vi "process_simple_input.vi"(10 "input line":string, 11 "RESP3 Parser in":refnum<class "RESP3 Parser.lvclass">) -> (0 "error out":errorcluster, 2 "value ready?":bool, 3 "RESP3 Parser out":refnum<class "RESP3 Parser.lvclass">, 4 "next bytes":i32)   [LabVIEW 2019, in "RESP3.lvlib" / "RESP3 Parser.lvclass"]
uses:
  RESP3 Parser.lvclass
  RESP3 Parser.lvclass/RESP3 Parser.ctl
  types/RESP3 Type.ctl
  RESP3.lvlib
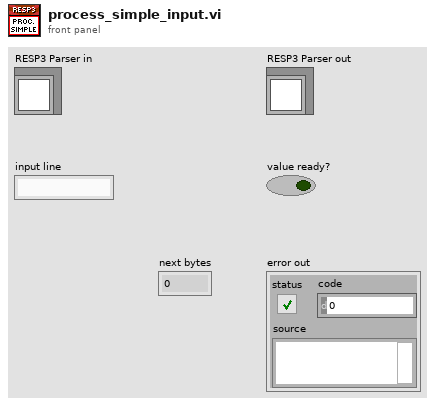
[diagram p1: front panel]
types:
  T1 = typedef "RESP3.lvlib/RESP3 Type.ctl" = enum8{"<0x00>", "<0x01>", "<0x02>", "<0x03>", "<0x04>", "<0x05>", "<0x06>", "<0x07>", "<0x08>", "<0x09>", "<0x0A>", "<0x0B>", "<0x0C>", "<0x0D>", "<0x0E>", "<0x0F>", "<0x10>", "<0x11>", "<0x12>", "<0x13>", "<0x14>", "<0x15>", "<0x16>", "<0x17>", "<0x18>", "<0x19>", "<0x1A>", "<0x1B>", "<0x1C>", "<0x1D>", "<0x1E>", "<0x1F>", "\" \"", "BLOB ERROR", "\"\"\"", "BOOLEAN", "BLOB", "MAP", "\"&\"", "\"'\"", "BIG NUMBER", "\")\"", "ARRAY", "STRING", "DOUBLE", "ERROR", "END", "\"/\"", "\"0\"", "\"1\"", "\"2\"", "\"3\"", "\"4\"", "\"5\"", "\"6\"", "\"7\"", "\"8\"", "\"9\"", "INTEGER", "STREAM", "\"<\"", "VERBATIM STRING", "PUSH", "\"?\"", "\"@\"", "\"A\"", "\"B\"", "\"C\"", "\"D\"", "\"E\"", "\"F\"", "\"G\"", "\"H\"", "\"I\"", "\"J\"", "\"K\"", "\"L\"", "\"M\"", "\"N\"", "\"O\"", "\"P\"", "\"Q\"", "\"R\"", "\"S\"", "\"T\"", "\"U\"", "\"V\"", "\"W\"", "\"X\"", "\"Y\"", "\"Z\"", "\"[\"", "\"\\\"", "\"]\"", "\"^\"", "NULL", "\"`\"", "\"a\"", "\"b\"", "\"c\"", "\"d\"", "\"e\"", "\"f\"", "\"g\"", "\"h\"", "\"i\"", "\"j\"", "\"k\"", "\"l\"", "\"m\"", "\"n\"", "\"o\"", "\"p\"", "\"q\"", "\"r\"", "\"s\"", "\"t\"", "\"u\"", "\"v\"", "\"w\"", "\"x\"", "\"y\"", "\"z\"", "\"{\"", "ATTRIBUTES", "\"}\"", "SET", "<0x7F>", "<0x80>", "<0x81>", "<0x82>", "<0x83>", "<0x84>", "<0x85>", "<0x86>", "<0x87>", "<0x88>", "<0x89>", "<0x8A>", "<0x8B>", "<0x8C>", "<0x8D>", "<0x8E>", "<0x8F>", "<0x90>", "<0x91>", "<0x92>", "<0x93>", "<0x94>", "<0x95>", "<0x96>", "<0x97>", "<0x98>", "<0x99>", "<0x9A>", "<0x9B>", "<0x9C>", "<0x9D>", "<0x9E>", "<0x9F>", "<0xA0>", "<0xA1>", "<0xA2>", "<0xA3>", "<0xA4>", "<0xA5>", "<0xA6>", "<0xA7>", "<0xA8>", "<0xA9>", "<0xAA>", "<0xAB>", "<0xAC>", "<0xAD>", "<0xAE>", "<0xAF>", "<0xB0>", "<0xB1>", "<0xB2>", "<0xB3>", "<0xB4>", "<0xB5>", "<0xB6>", "<0xB7>", "<0xB8>", "<0xB9>", "<0xBA>", "<0xBB>", "<0xBC>", "<0xBD>", "<0xBE>", "<0xBF>", "<0xC0>", "<0xC1>", "<0xC2>", "<0xC3>", "<0xC4>", "<0xC5>", "<0xC6>", "<0xC7>", "<0xC8>", "<0xC9>", "<0xCA>", "<0xCB>", "<0xCC>", "<0xCD>", "<0xCE>", "<0xCF>", "<0xD0>", "<0xD1>", "<0xD2>", "<0xD3>", "<0xD4>", "<0xD5>", "<0xD6>", "<0xD7>", "<0xD8>", "<0xD9>", "<0xDA>", "<0xDB>", "<0xDC>", "<0xDD>", "<0xDE>", "<0xDF>", "<0xE0>", "<0xE1>", "<0xE2>", "<0xE3>", "<0xE4>", "<0xE5>", "<0xE6>", "<0xE7>", "<0xE8>", "<0xE9>", "<0xEA>", "<0xEB>", "<0xEC>", "<0xED>", "<0xEE>", "<0xEF>", "<0xF0>", "<0xF1>", "<0xF2>", "<0xF3>", "<0xF4>", "<0xF5>", "<0xF6>", "<0xF7>", "<0xF8>", "<0xF9>", "<0xFA>", "<0xFB>", "<0xFC>", "<0xFD>", "<0xFE>"}
  T2 = cluster{"index":i32, "remaining elements":i32, "nest type":T1}[]
  T3 = cluster{"index":i32, "remaining elements":i32, "char":T1}[]
  T4 = cluster{"index":i32, "remaining elements":i32, "nest type":T1}
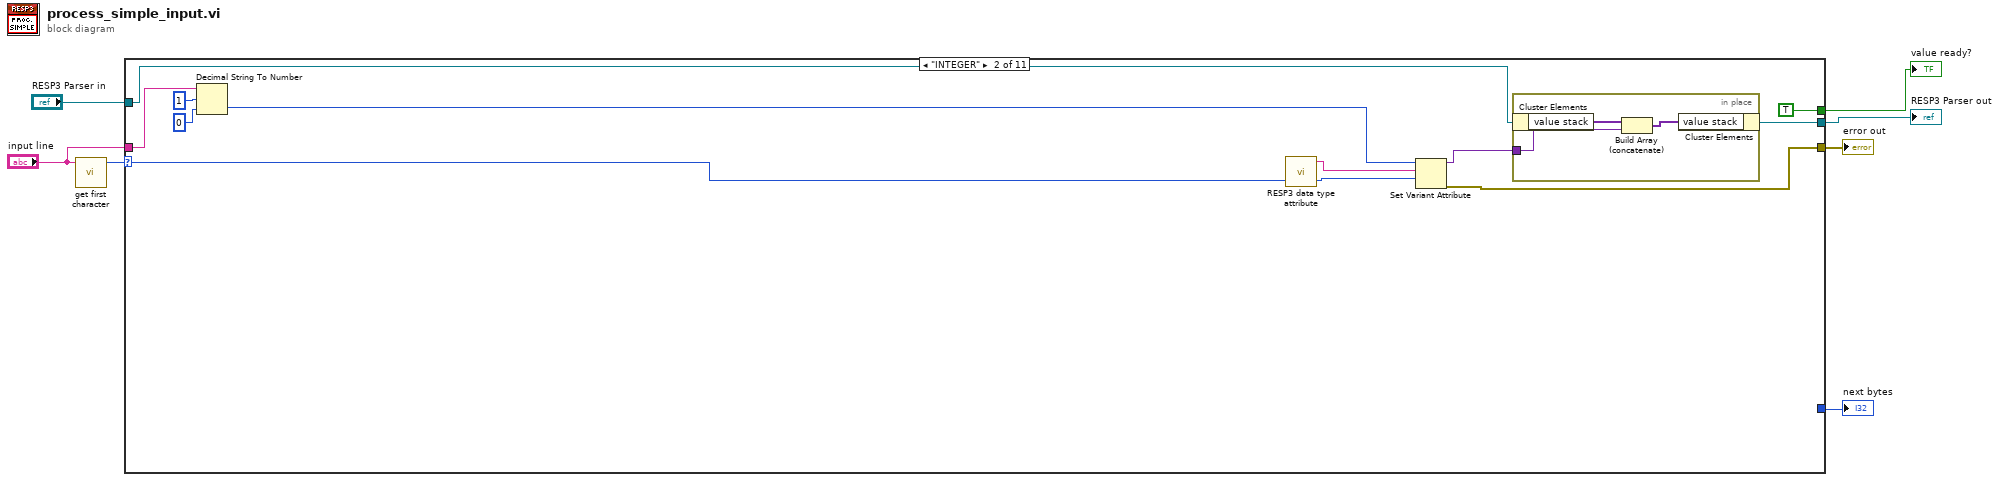
[diagram p0: block diagram]
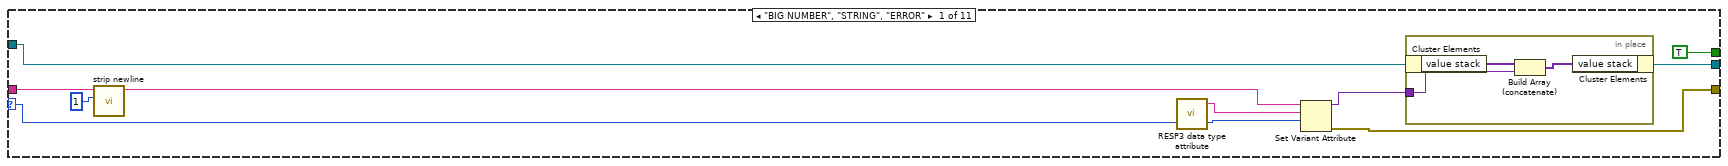
[diagram p2: hidden frame]
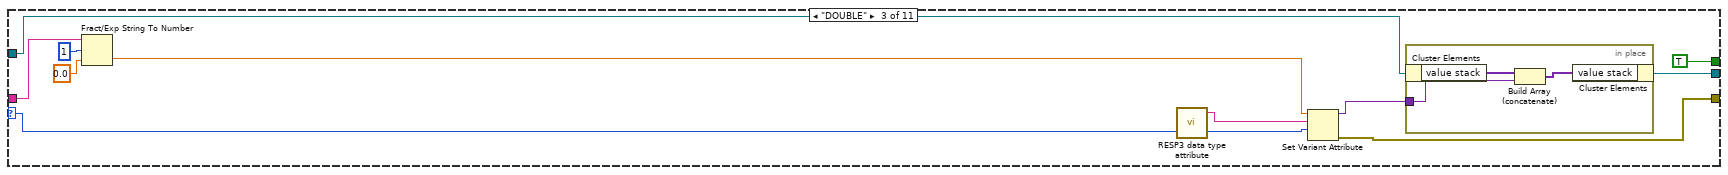
[diagram p3: hidden frame]
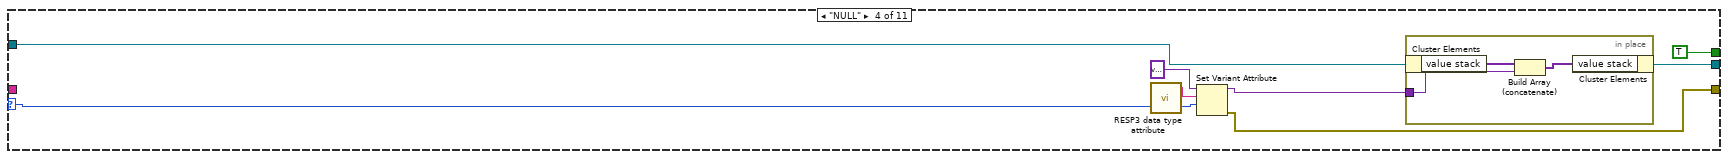
[diagram p4: hidden frame]
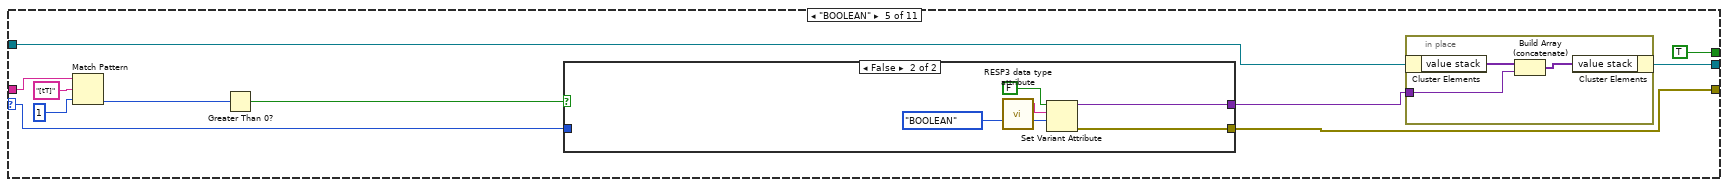
[diagram p5: hidden frame]
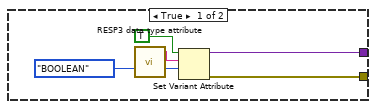
[diagram p6: hidden frame]
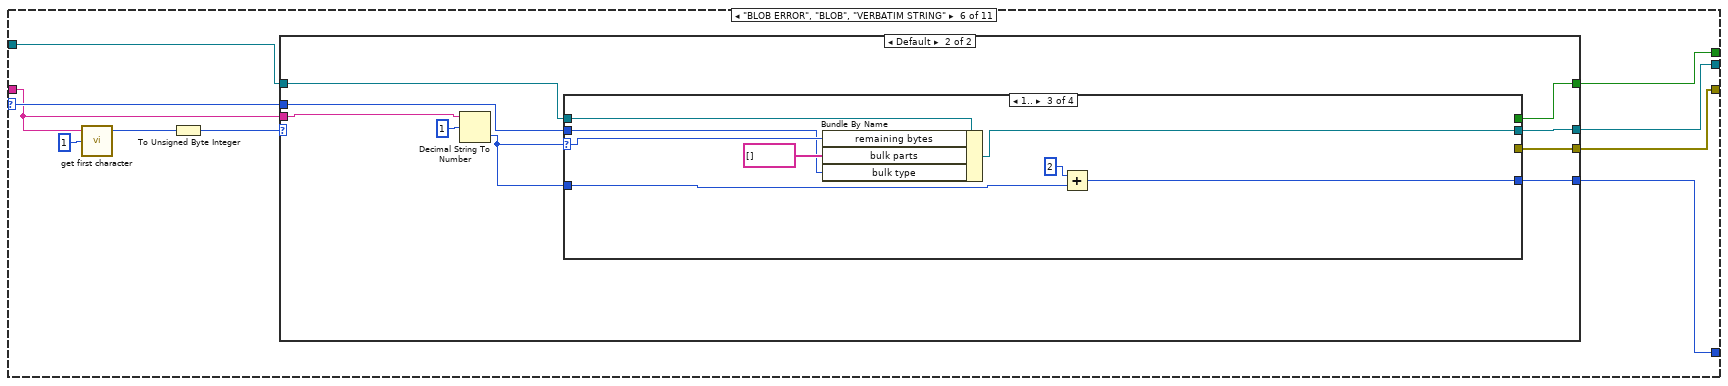
[diagram p7: hidden frame]
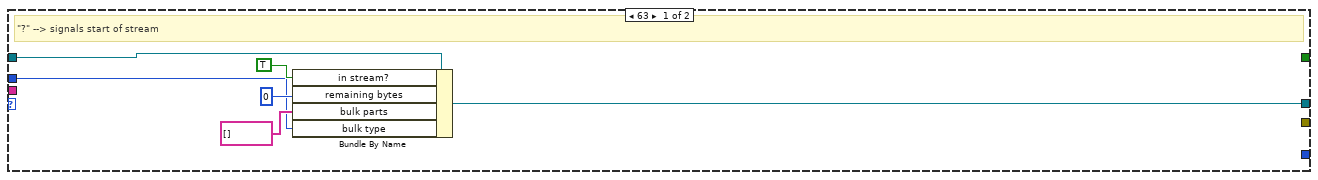
[diagram p8: hidden frame]
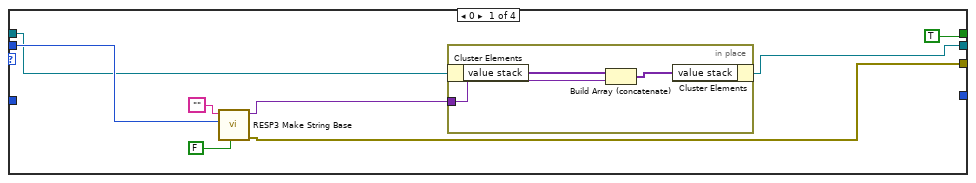
[diagram p9: hidden frame]
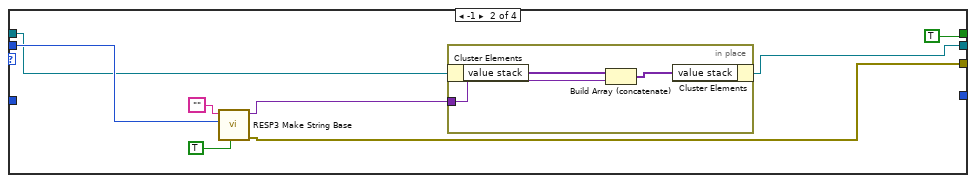
[diagram p10: hidden frame]
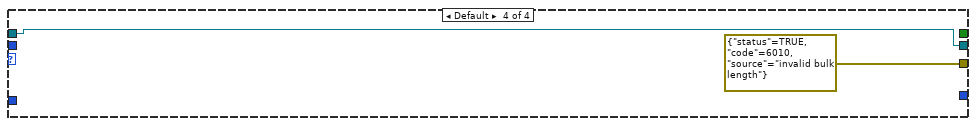
[diagram p11: hidden frame]
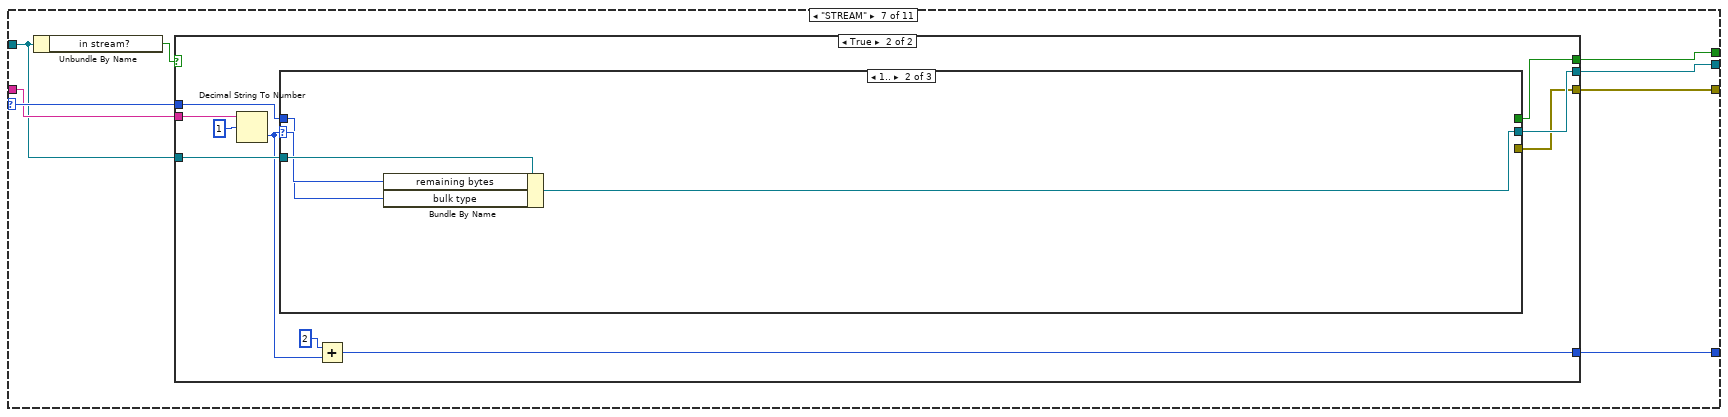
[diagram p12: hidden frame]
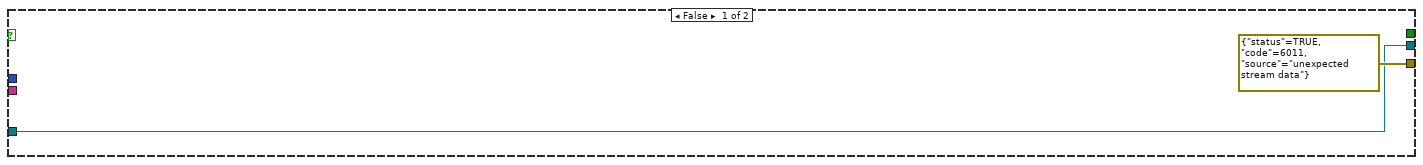
[diagram p13: hidden frame]
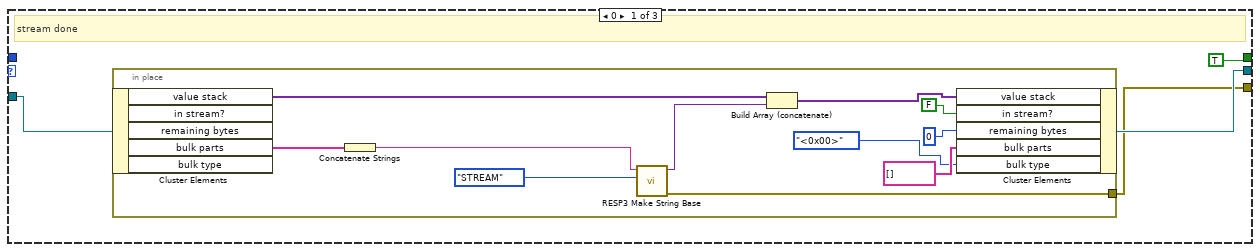
[diagram p14: hidden frame]
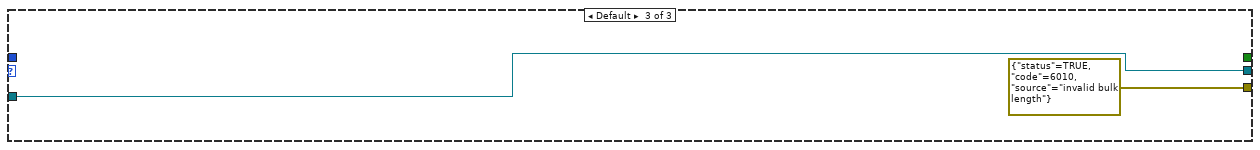
[diagram p15: hidden frame]
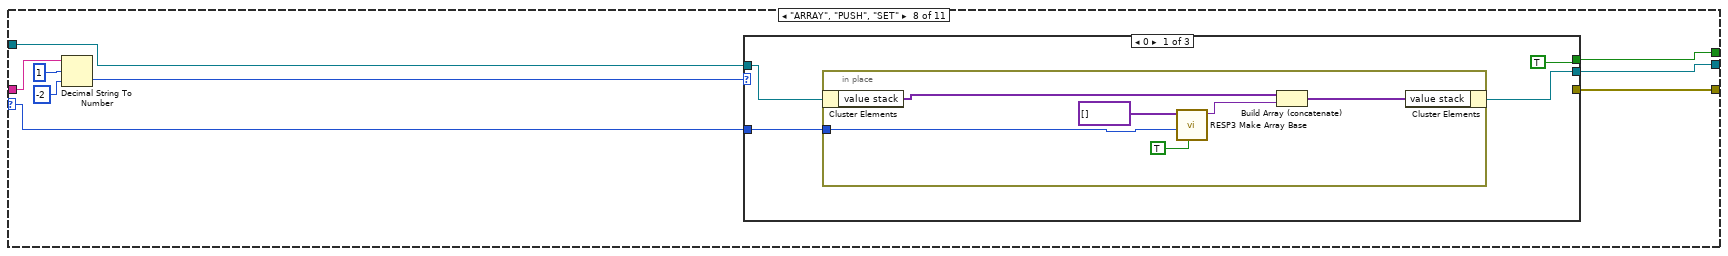
[diagram p16: hidden frame]
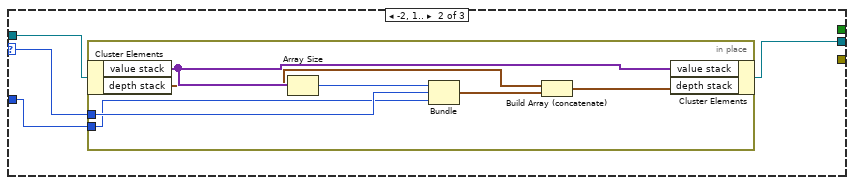
[diagram p17: hidden frame]
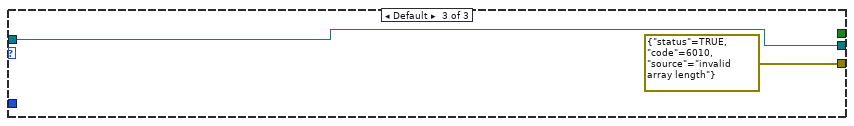
[diagram p18: hidden frame]
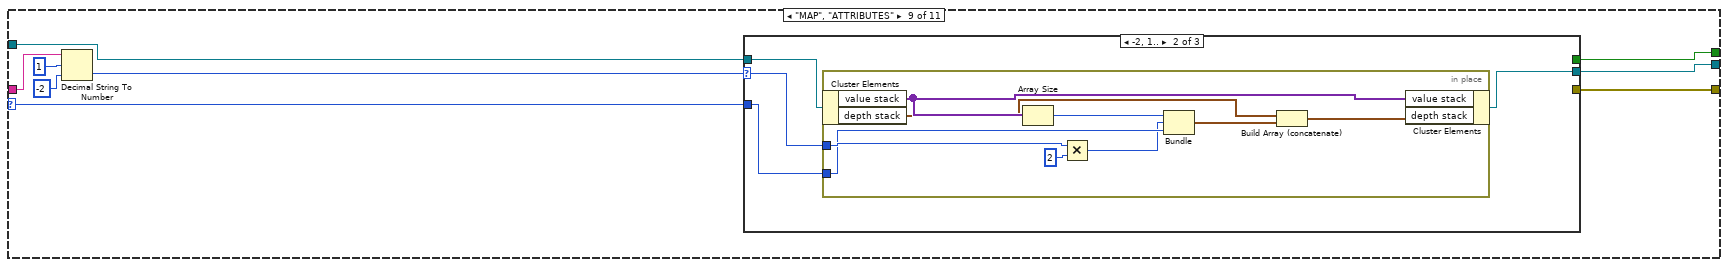
[diagram p19: hidden frame]
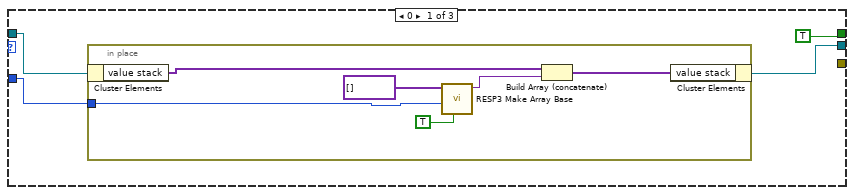
[diagram p20: hidden frame]
diagram:
  n1 = call "get first character.vi"("input"="input line") -> ("char"=w2:T1)  [unwired: 4 in]
  n2 = case shown="\"INTEGER\"" w2 {
    selector: w2 -> [w9 w26 w40 w51 w66 w91 w147 w183 w215 _ _]
    tunnel: "input line" -> [w17 w24 w38 _ w64 w89 w145 w190 w222 _ _]
    tunnel: [TRUE TRUE TRUE TRUE TRUE w85 w144 w185 w217 w249 _] -> w3
    tunnel: "RESP3 Parser in" -> [w14 w30 w44 w55 w69 w93 w143 w188 w220 w250 w265]
    tunnel: [w13 w29 w43 w54 w68 w92 w148 w187 w219 w248 w265] -> w4
    tunnel: [w8 w25 w39 w50 w65 w90 w146 w184 w216 _ _] -> w7
    tunnel: [_ _ _ _ _ w84 w141 _ _ _ _] -> w1
    frame "BIG NUMBER", "STRING", "ERROR" {
      n3 = call "strip newline.vi"("offset"=1, "\\r\\n terminated string"=w17) -> ("striped string"=w12:string)  [unwired: 9 in]
      n4 = call "RESP3 data type attribute.vi"() -> ("dt attribute"=w10:string)  [unwired: 5 in]
      n5 = Set Variant Attribute(Variant=w12, name=w10, value=w9) -> (Variant out=w11:variant, error out=w8:errorcluster)  [unwired: 1 in, 1 out]
      n6 = in-place {
        in-place-border: w11 -> [w19]
        n7 = in-place-cluster #1(w14) -> ("value stack"=w20:variant[])
        n8 = Build Array (concatenate)(w20, w19) -> (w18:variant[])
        n9 = in-place-cluster #1("value stack"=w18) -> (w13:refnum<class "RESP3 Parser.lvclass">)
      }
    }
    frame "INTEGER" {
      n10 = Decimal String To Number(string=w24, offset=1, default (0L)=i64 0 ("default (0 I32)")) -> (number=w21:i64)  [unwired: 1 out]
      n11 = call "RESP3 data type attribute.vi"() -> ("dt attribute"=w27:string)  [unwired: 5 in]
      n12 = Set Variant Attribute(Variant=w21, name=w27, value=w26) -> (Variant out=w28:variant, error out=w25:errorcluster)  [unwired: 1 in, 1 out]
      n13 = in-place {
        in-place-border: w28 -> [w33]
        n14 = in-place-cluster #2(w30) -> ("value stack"=w34:variant[])
        n15 = Build Array (concatenate)(w34, w33) -> (w32:variant[])
        n16 = in-place-cluster #2("value stack"=w32) -> (w29:refnum<class "RESP3 Parser.lvclass">)
      }
    }
    frame "DOUBLE" {
      n17 = Fract/Exp String To Number(string=w38, offset=1, default (0 dbl)=0.0 ("default (0 I32)")) -> (number=w35:dbl)  [unwired: 1 in, 1 out]
      n18 = call "RESP3 data type attribute.vi"() -> ("dt attribute"=w41:string)  [unwired: 5 in]
      n19 = Set Variant Attribute(Variant=w35, name=w41, value=w40) -> (Variant out=w42:variant, error out=w39:errorcluster)  [unwired: 1 in, 1 out]
      n20 = in-place {
        in-place-border: w42 -> [w47]
        n21 = in-place-cluster #3(w44) -> ("value stack"=w48:variant[])
        n22 = Build Array (concatenate)(w48, w47) -> (w46:variant[])
        n23 = in-place-cluster #3("value stack"=w46) -> (w43:refnum<class "RESP3 Parser.lvclass">)
      }
    }
    frame "NULL" {
      n24 = call "RESP3 data type attribute.vi"() -> ("dt attribute"=w52:string)  [unwired: 5 in]
      n25 = Set Variant Attribute(Variant=variant, name=w52, value=w51) -> (Variant out=w53:variant, error out=w50:errorcluster)  [unwired: 1 in, 1 out]
      n26 = in-place {
        in-place-border: w53 -> [w58]
        n27 = in-place-cluster #4(w55) -> ("value stack"=w59:variant[])
        n28 = Build Array (concatenate)(w59, w58) -> (w57:variant[])
        n29 = in-place-cluster #4("value stack"=w57) -> (w54:refnum<class "RESP3 Parser.lvclass">)
      }
    }
    frame "BOOLEAN" {
      n30 = Match Pattern(string=w64, regular expression="[tT]", offset (0)=1) -> (offset past match=w61:i32)  [unwired: 3 out]
      n31 = Greater Than 0?(x=w61) -> (x > 0?=w60:bool)
      n32 = case shown="False" w60 {
        tunnel: [w75 w80] -> w67
        tunnel: w66 -> [_ _]
        tunnel: [w73 w78] -> w65
        frame True {
          n33 = call "RESP3 data type attribute.vi"() -> ("dt attribute"=w74:string)  [unwired: 5 in]
          n34 = Set Variant Attribute(Variant=TRUE, name=w74, value=RESP3_Type."BOOLEAN" ("char")) -> (Variant out=w75:variant, error out=w73:errorcluster)  [unwired: 1 in, 1 out]
        }
        frame False {
          n35 = call "RESP3 data type attribute.vi"() -> ("dt attribute"=w79:string)  [unwired: 5 in]
          n36 = Set Variant Attribute(Variant=FALSE, name=w79, value=RESP3_Type."BOOLEAN" ("char")) -> (Variant out=w80:variant, error out=w78:errorcluster)  [unwired: 1 in, 1 out]
        }
      }
      n37 = in-place {
        in-place-border: w67 -> [w82]
        n38 = in-place-cluster #5(w69) -> ("value stack"=w83:variant[])
        n39 = Build Array (concatenate)(w83, w82) -> (w81:variant[])
        n40 = in-place-cluster #5("value stack"=w81) -> (w68:refnum<class "RESP3 Parser.lvclass">)
      }
    }
    frame "BLOB ERROR", "BLOB", "VERBATIM STRING" {
      n41 = call "get first character.vi"("index"=1, "input"=w89) -> ("char"=w87:T1)  [unwired: 3 in]
      n42 = To Unsigned Byte Integer(number=w87) -> (unsigned 8bit integer=w86:u8)
      n43 = case shown="Default" w86 {
        tunnel: w93 -> [w99 w107]
        tunnel: [w98 w106] -> w92
        tunnel: w91 -> [w94 w105]
        tunnel: [_ w104] -> w90
        tunnel: w89 -> [_ w103]
        tunnel: [_ w102] -> w85
        tunnel: [_ w100] -> w84
        frame 63 {
          # "\"?\" --> signals start of stream"
          n44 = Bundle By Name(cluster=w99, "in stream?"=TRUE ("bulk data.in stream?"), "remaining bytes"=0 ("bulk data.remaining bytes"), "bulk parts"=string[] [] ("bulk data.bulk parts"), "bulk type"=w94) -> (w98:refnum<class "RESP3 Parser.lvclass">)
        }
        frame Default {
          n45 = Decimal String To Number(string=w103, offset=1) -> (number=w101:i32)  [unwired: 1 in, 1 out]
          n46 = case shown="1.." w101 {
            selector: w101 -> [_ _ w135 _]
            tunnel: w107 -> [w113 w124 w137 w139]
            tunnel: [w116 w127 w136 w139] -> w106
            tunnel: w105 -> [w115 w126 w134 _]
            tunnel: [w114 w125 _ errorcluster {"status"=TRUE, "code"=6010, "source"="invalid bulk length"} ("error out")] -> w104
            tunnel: [TRUE TRUE _ _] -> w102
            tunnel: w101 -> [_ _ w133 _]
            tunnel: [_ _ w131 _] -> w100
            frame 0 {
              n47 = call "RESP3 Make String Base.vi"("is null?"=FALSE, "RESP3 String Type"=w115, "string in"="") -> ("error out"=w114:errorcluster, "RESP3 Value out"=w109:variant)  [unwired: 7 in]
              n48 = in-place {
                in-place-border: w109 -> [w117]
                n49 = in-place-cluster #6(w113) -> ("value stack"=w119:variant[])
                n50 = Build Array (concatenate)(w119, w117) -> (w118:variant[])
                n51 = in-place-cluster #6("value stack"=w118) -> (w116:refnum<class "RESP3 Parser.lvclass">)
              }
            }
            frame -1 {
              n52 = call "RESP3 Make String Base.vi"("is null?"=TRUE, "RESP3 String Type"=w126, "string in"="") -> ("error out"=w125:errorcluster, "RESP3 Value out"=w120:variant)  [unwired: 7 in]
              n53 = in-place {
                in-place-border: w120 -> [w128]
                n54 = in-place-cluster #7(w124) -> ("value stack"=w130:variant[])
                n55 = Build Array (concatenate)(w130, w128) -> (w129:variant[])
                n56 = in-place-cluster #7("value stack"=w129) -> (w127:refnum<class "RESP3 Parser.lvclass">)
              }
            }
            frame 1.. {
              n57 = Bundle By Name(cluster=w137, "remaining bytes"=w135, "bulk parts"=string[] [] ("bulk data.bulk parts"), "bulk type"=w134) -> (w136:refnum<class "RESP3 Parser.lvclass">)
              n58 = Add(x=2, y=w133) -> (x+y=w131:i32)
            }
            frame Default {
            }
          }
        }
      }
    }
    frame "STREAM" {
      n59 = Unbundle By Name(w143) -> ("in stream?"=w142:bool)
      n60 = case shown="True" w142 {
        tunnel: [w149 w160] -> w148
        tunnel: w147 -> [_ w159]
        tunnel: [errorcluster {"status"=TRUE, "code"=6011, "source"="unexpected stream data"} ("error out") w158] -> w146
        tunnel: w145 -> [_ w157]
        tunnel: [_ w156] -> w144
        tunnel: w143 -> [w149 w154]
        tunnel: [_ w152] -> w141
        frame False {
        }
        frame True {
          n61 = Decimal String To Number(string=w157, offset=1) -> (number=w153:i32)  [unwired: 1 in, 1 out]
          n62 = case shown="1.." w153 {
            selector: w153 -> [_ w177 _]
            tunnel: w154 -> [w163 w179 w180]
            tunnel: [w162 w178 w180] -> w160
            tunnel: w159 -> [_ w176 _]
            tunnel: [w161 _ errorcluster {"status"=TRUE, "code"=6010, "source"="invalid bulk length"} ("error out")] -> w158
            tunnel: [TRUE _ _] -> w156
            frame 0 {
              # "stream done"
              n63 = in-place {
                in-place-border: [w165] -> w161
                n64 = in-place-cluster #8(w163) -> ("value stack"=w175:variant[], "bulk parts"=w167:string[])  [unwired: 3 out]
                n65 = Concatenate Strings(w167) -> (w166:string)
                n66 = call "RESP3 Make String Base.vi"("RESP3 String Type"=RESP3_Type."STREAM", "string in"=w166) -> ("error out"=w165:errorcluster, "RESP3 Value out"=w173:variant)  [unwired: 8 in]
                n67 = Build Array (concatenate)(w175, w173) -> (w174:variant[])
                n68 = in-place-cluster #8("value stack"=w174, "in stream?"=FALSE ("bulk data.in stream?"), "remaining bytes"=0 ("bulk data.remaining bytes"), "bulk parts"=string[] [] ("bulk data.bulk parts"), "bulk type"=RESP3_Type."<0x00>" ("bulk data.bulk type")) -> (w162:refnum<class "RESP3 Parser.lvclass">)
              }
            }
            frame 1.. {
              n69 = Bundle By Name(cluster=w179, "remaining bytes"=w177, "bulk type"=w176) -> (w178:refnum<class "RESP3 Parser.lvclass">)
            }
            frame Default {
            }
          }
          n70 = Add(x=2, y=w153) -> (x+y=w152:i32)
        }
      }
    }
    frame "ARRAY", "PUSH", "SET" {
      n71 = Decimal String To Number(string=w190, offset=1, default (0L)=-2 ("default (0 I32)")) -> (number=w186:i32)  [unwired: 1 out]
      n72 = case shown="0" w186 {
        selector: w186 -> [_ w202 _]
        tunnel: w188 -> [w194 w204 w213]
        tunnel: [w193 w203 w213] -> w187
        tunnel: [TRUE _ _] -> w185
        tunnel: [_ _ errorcluster {"status"=TRUE, "code"=6010, "source"="invalid array length"} ("error out")] -> w184
        tunnel: w183 -> [w191 w201 _]
        frame 0 {
          n73 = in-place {
            in-place-border: w191 -> [w195]
            n74 = in-place-cluster #9(w194) -> ("value stack"=w200:variant[])
            n75 = call "RESP3 Make Array Base.vi"("is null?"=TRUE, "RESP3 Type"=w195, "RESP3 Values in"=variant[] []) -> ("RESP3 Value out"=w196:variant)  [unwired: 7 in, 1 out]
            n76 = Build Array (concatenate)(w200, w196) -> (w199:variant[])
            n77 = in-place-cluster #9("value stack"=w199) -> (w193:refnum<class "RESP3 Parser.lvclass">)
          }
        }
        frame -2, 1.. {
          n78 = in-place {
            in-place-border: w202 -> [w207]
            in-place-border: w201 -> [w205]
            n79 = in-place-cluster #10(w204) -> ("value stack"=w211:variant[], "depth stack"=w210:T2)
            n80 = Array Size(array=w211) -> (size(s)=w208:i32)
            n81 = Bundle(w208, w207, "char"=w205) -> (w206:cluster{i32, i32, "char":T1})  [unwired: 1 in]
            n82 = Build Array (concatenate)(w210, w206) -> (w209:T3)
            n83 = in-place-cluster #10("value stack"=w211, "depth stack"=w209) -> (w203:refnum<class "RESP3 Parser.lvclass">)
          }
        }
        frame Default {
        }
      }
    }
    frame "MAP", "ATTRIBUTES" {
      n84 = Decimal String To Number(string=w222, offset=1, default (0L)=-2 ("default (0 I32)")) -> (number=w218:i32)  [unwired: 1 out]
      n85 = case shown="-2, 1.." w218 {
        selector: w218 -> [_ w234 _]
        tunnel: w220 -> [w226 w236 w247]
        tunnel: [w225 w235 w247] -> w219
        tunnel: [TRUE _ _] -> w217
        tunnel: [_ _ errorcluster {"status"=TRUE, "code"=6010, "source"="invalid array length"} ("error out")] -> w216
        tunnel: w215 -> [w223 w233 _]
        frame 0 {
          n86 = in-place {
            in-place-border: w223 -> [w227]
            n87 = in-place-cluster #11(w226) -> ("value stack"=w232:variant[])
            n88 = call "RESP3 Make Array Base.vi"("is null?"=TRUE, "RESP3 Type"=w227, "RESP3 Values in"=variant[] []) -> ("RESP3 Value out"=w228:variant)  [unwired: 7 in, 1 out]
            n89 = Build Array (concatenate)(w232, w228) -> (w231:variant[])
            n90 = in-place-cluster #11("value stack"=w231) -> (w225:refnum<class "RESP3 Parser.lvclass">)
          }
        }
        frame -2, 1.. {
          n91 = in-place {
            in-place-border: w234 -> [w241]
            in-place-border: w233 -> [w239]
            n92 = in-place-cluster #12(w236) -> ("value stack"=w245:variant[], "depth stack"=w244:T2)
            n93 = Array Size(array=w245) -> (size(s)=w242:i32)
            n94 = Multiply(x=w241, y=2) -> (x*y=w238:i32)
            n95 = Bundle(w242, w238, "char"=w239) -> (w240:cluster{i32, i32, "char":T1})  [unwired: 1 in]
            n96 = Build Array (concatenate)(w244, w240) -> (w243:T3)
            n97 = in-place-cluster #12("value stack"=w245, "depth stack"=w243) -> (w235:refnum<class "RESP3 Parser.lvclass">)
          }
        }
        frame Default {
        }
      }
    }
    frame "END" {
      n98 = in-place {
        in-place-border: [w251] -> w249
        n99 = in-place-cluster #13(w250) -> ("depth stack"=w252:T2)
        n100 = Array Size(array=w252) -> (size(s)=w254:i32)
        n101 = case shown="1.." w254 {
          selector: w254 -> [w258 _]
          tunnel: [w256 w264] -> w253
          tunnel: w252 -> [w259 w264]
          tunnel: [w255 _] -> w251
          frame 1.. {
            n102 = Decrement(x=w258) -> (x-1=w257:i32)
            n103 = in-place {
              in-place-border: [TRUE] -> w255
              n104 = in-place-array #14(w259, w257) -> (w263:T4)
              n105 = Bundle By Name(cluster=w263, "remaining elements"=1) -> (w261:T4)
              n106 = in-place-array #14(w261) -> (w256:T2)  [unwired: 1 out]
            }
          }
          frame ..0 {
          }
        }
        n107 = in-place-cluster #13("depth stack"=w253) -> (w248:refnum<class "RESP3 Parser.lvclass">)
      }
    }
    frame Default {
    }
  }
  "error out" <- w7
  "RESP3 Parser out" <- w4
  "value ready?" <- w3
  "next bytes" <- w1
